vi "Command Voltage Limit.vi"(2 "error in (no error)":errorcluster, 3 "ID":T3) -> (0 "error out":errorcluster)   [LabVIEW 2009]
uses:
  lib/Data Access Objects/Metadata/LBCB Number.ctl
  lib/Data Access Objects/Metadata/Actuator Matrix.ctl
  lib/Data Access Objects/Metadata/Actuator Point.ctl
  Update Actions.ctl
  lib/Data Access Objects/Metadata/Persistant DAO Actions.ctl
panel:
  out "L2 Command Voltage Limit Default":T1
  out "L1 Command Voltage Limit Default":T1
  in  "Command Voltage Limit":dbl[][](array[numeric])=[[-9.5, -9.5], [-9.5, 9.5], [-9.5, 9.5], [-9.5, 9.5], [-9.5, 9.5], [-9.5, 9.5]]
  in  "Cancel":bool
  in  "OK":bool
  # "Command\nVoltage \nLimit"
  # "Lower\n(V)"
  # "Upper\n(V)"
  # "Actuator X1"
  # "Actuator X2"
  # "Actuator Y1"
  # "Actuator Z1"
  # "Actuator Z2"
  # "Actuator Z3"
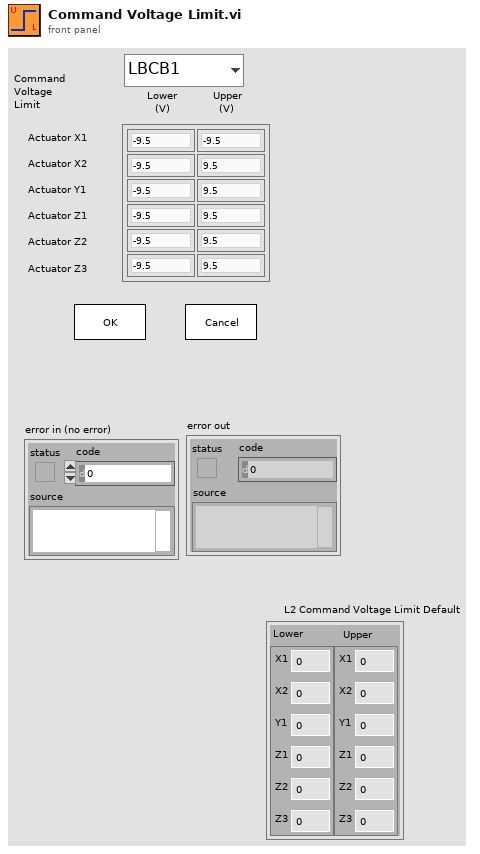
[diagram p1: front panel]
types:
  T1 = typedef "Actuator Matrix.ctl" = cluster{"Lower":T2, "Upper":T2}
  T2 = typedef "Actuator Point.ctl" = cluster{"X1":dbl, "X2":dbl, "Y1":dbl, "Z1":dbl, "Z2":dbl, "Z3":dbl}
  T3 = typedef "LBCB Number.ctl" = enum16{"LBCB1", "LBCB2"}
  T4 = typedef "Persistant DAO Actions.ctl" = enum16{"Init", "Get", "Set", "Load", "Save"}
  T5 = typedef "Update Actions.ctl" = enum16{"Update", "Exit"}
  T6 = typedef "Limit Matrix.ctl" = dbl[][]
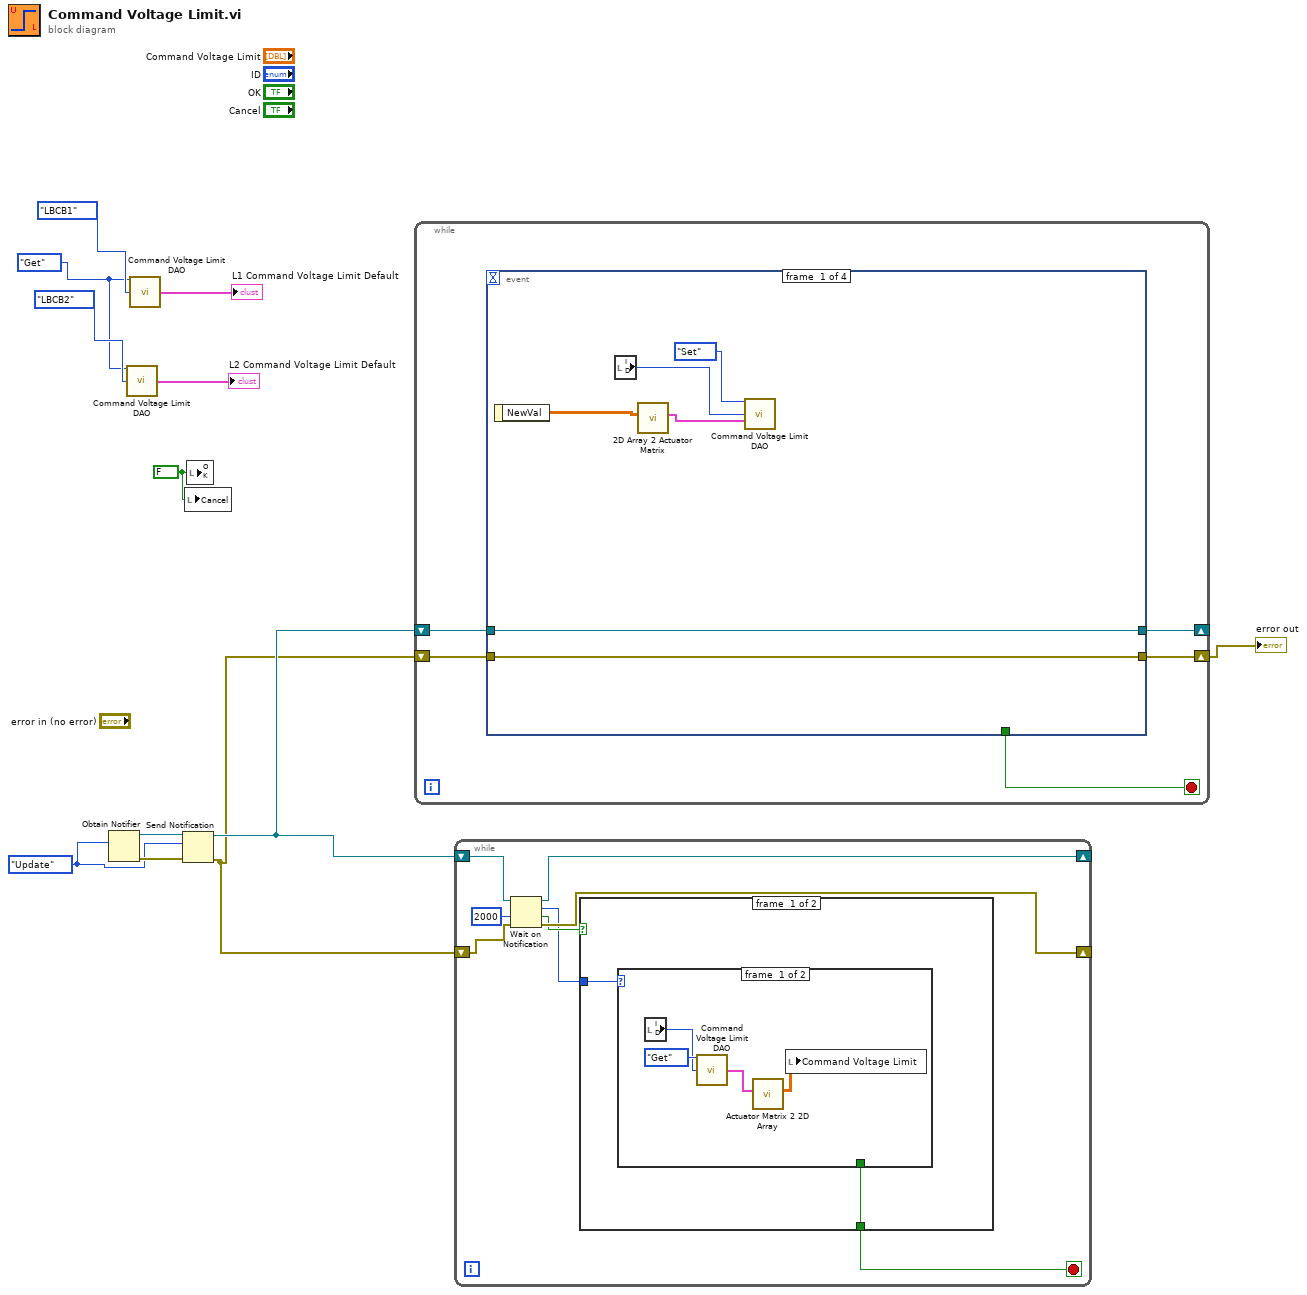
[diagram p0: block diagram]
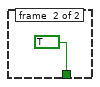
[diagram p2: hidden frame]
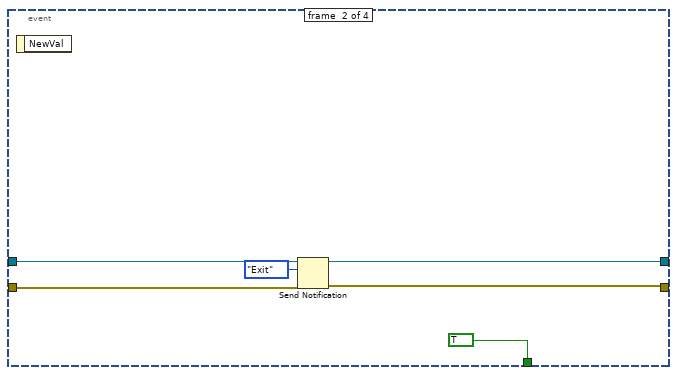
[diagram p4: hidden frame]
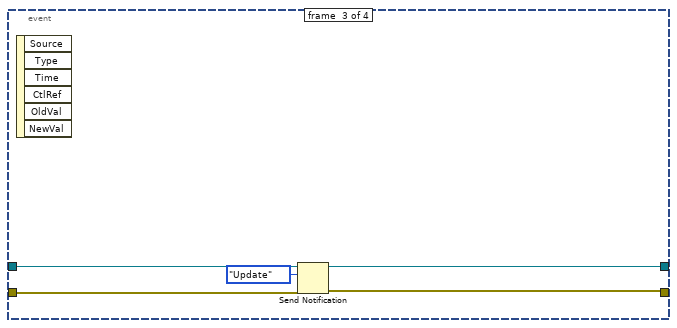
[diagram p5: hidden frame]
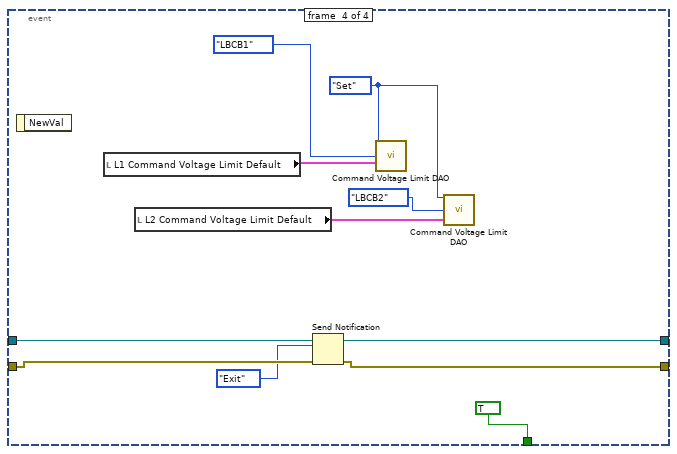
[diagram p6: hidden frame]
diagram:
  w1 = FALSE ("OK")
  w5 = Persistant_DAO_Actions."Get" ("Actuator Stroke Limit Actions")
  w10 = Update_Actions."Update" ("Update Actions")
  n1 = Obtain Notifier(notification data type=w10) -> (notifier out=w11:refnum<notifier>, error out=w12:errorcluster)  [unwired: 2 in, 2 out]
  n2 = call "Command Voltage Limit DAO.vi"("Actuator Stroke Limit Actions"=w5, "ID"=LBCB_Number."LBCB2") -> ("Command Voltage Limit Out"=→"L2 Command Voltage Limit Default":T1)  [unwired: 3 in, 10 out]
  n3 = call "Command Voltage Limit DAO.vi"("Actuator Stroke Limit Actions"=w5, "ID"=LBCB_Number."LBCB1") -> ("Command Voltage Limit Out"=→"L1 Command Voltage Limit Default":T1)  [unwired: 3 in, 10 out]
  n4 = Send Notification(notification=w10, notifier=w11, error in (no error)=w12) -> (notifier out=w4:refnum<notifier>, error out=w3:errorcluster)
  n5 = local write "Cancel"(w1) -> ()
  n6 = local write "OK"(w1) -> ()
  n7 = while {
    shift-right: [w13] -> _
    shift-left: w4 -> [w16]
    shift-right: [w14] -> w2
    shift-left: w3 -> [w15]
    stop <- w17 stop-if-true
    n8 = event shown="[3] \"Cancel\": Value Change" {
      selector: _ -> [_ _ _ _]
      dyn-events: _ -> [_ _ _ _]
      timeout: _ -> [_ _ _ _]
      tunnel: [_ TRUE _ TRUE] -> w17
      tunnel: w16 -> [w19 w28 w34 w40]
      tunnel: w15 -> [w18 w26 w32 w39]
      tunnel: [w18 w25 w31 w37] -> w14
      tunnel: [w19 w27 w33 w38] -> w13
      event #0 {
        n9 = event-data() -> ("NewVal"=w23:dbl[][])  [unwired: 1 out]
        n10 = local read "ID"() -> (w20:T3)
        n11 = call "2D Array 2 Actuator Matrix.vi"("Matrix In"=w23) -> ("Matrix Out"=w22:T1)  [unwired: 10 out]
        n12 = call "Command Voltage Limit DAO.vi"("Actuator Stroke Limit Actions"=Persistant_DAO_Actions."Set", "ID"=w20, "Command Voltage Limit In"=w22) -> ()  [unwired: 2 in, 11 out]
      }
      event #1 {
        n13 = event-data() -> ()  [unwired: 2 out]
        n14 = Send Notification(notification=Update_Actions."Exit", notifier=w28, error in (no error)=w26) -> (notifier out=w27:refnum<notifier>, error out=w25:errorcluster)
      }
      event #2 {
        n15 = event-data() -> ()  [unwired: 7 out]
        n16 = Send Notification(notification=Update_Actions."Update", notifier=w34, error in (no error)=w32) -> (notifier out=w33:refnum<notifier>, error out=w31:errorcluster)
      }
      event #3 {
        w43 = Persistant_DAO_Actions."Set" ("Actuator Stroke Limit Actions")
        n17 = event-data() -> ()  [unwired: 2 out]
        n18 = local read "L1 Command Voltage Limit Default"() -> (w45:T1)
        n19 = local read "L2 Command Voltage Limit Default"() -> (w42:T1)
        n20 = Send Notification(notification=Update_Actions."Exit", notifier=w40, error in (no error)=w39) -> (notifier out=w38:refnum<notifier>, error out=w37:errorcluster)
        n21 = call "Command Voltage Limit DAO.vi"("Actuator Stroke Limit Actions"=w43, "ID"=LBCB_Number."LBCB1", "Command Voltage Limit In"=w45) -> ()  [unwired: 2 in, 11 out]
        n22 = call "Command Voltage Limit DAO.vi"("Actuator Stroke Limit Actions"=w43, "ID"=LBCB_Number."LBCB2", "Command Voltage Limit In"=w42) -> ()  [unwired: 2 in, 11 out]
      }
    }
  }
  "error out" <- w2
  n23 = while {
    shift-right: [w49] -> _
    shift-left: w3 -> [w52]
    shift-right: [w50] -> _
    shift-left: w4 -> [w51]
    stop <- w46 stop-if-true
    n24 = Wait on Notification(notifier=w51, timeout in ms (-1)=2000, error in (no error)=w52) -> (notifier out=w50:refnum<notifier>, notification=w47:T5, timed out?=w48:bool, error out=w49:errorcluster)  [unwired: 1 out]
    n25 = case shown="False" w48 {
      tunnel: w47 -> [w55 _]
      tunnel: [w54 _] -> w46
      frame #0 {
        n26 = case shown="\"Update\"" w55 {
          tunnel: [_ TRUE] -> w54
          frame #0 {
            n27 = local read "ID"() -> (w56:T3)
            n28 = call "Command Voltage Limit DAO.vi"("Actuator Stroke Limit Actions"=Persistant_DAO_Actions."Get", "ID"=w56) -> ("Command Voltage Limit Out"=w58:T1)  [unwired: 3 in, 10 out]
            n29 = call "Actuator Matrix 2 2D Array.vi"("Matrix In"=w58) -> ("Matrix Out"=w57:T6)  [unwired: 10 out]
            n30 = local write "Command Voltage Limit"(w57) -> ()
          }
          frame #1 {
          }
        }
      }
      frame #1 {
      }
    }
  }
